vi "CumplimientoTD.vi"(8 "error in (no error)":errorcluster, 11 "Prueba21_1 in":refnum<class "Prueba21.lvclass">) -> (0 "error out":errorcluster, 3 "Prueba21_1 out":refnum<class "Prueba21.lvclass">)   [LabVIEW 2019, in "Prueba21.lvclass"]
uses:
  Prueba21.lvclass
  Prueba21.lvclass/Prueba21.ctl
panel:
  out "cumpimiento":string
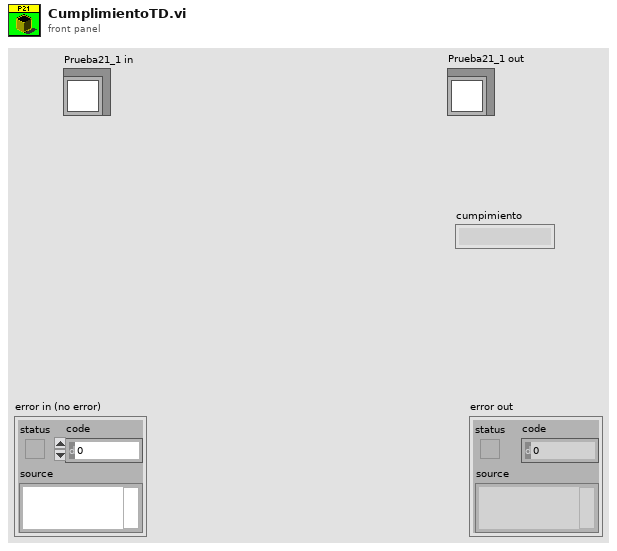
[diagram p1: front panel]
types:
  T1 = cluster{"ControlName":string, "ControlReference":refnum<vi>}[]
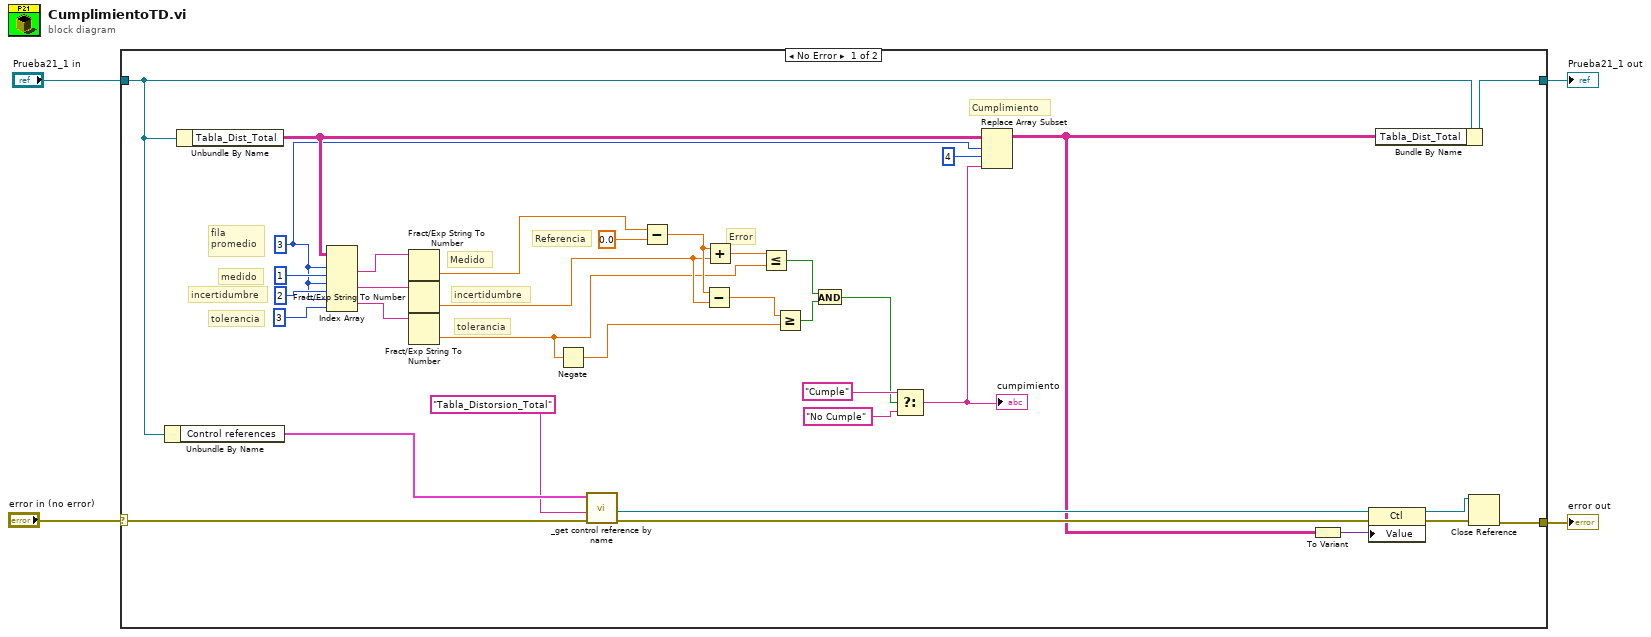
[diagram p0: block diagram]
diagram:
  n1 = case shown="No Error" "error in (no error)" {
    selector: "error in (no error)" -> [w11 w41]
    tunnel: [w13 w41] -> w3
    tunnel: [w30 w40] -> w2
    tunnel: "Prueba21_1 in" -> [w20 w40]
    frame No Error {
      w25 = 3 ("index (row)")
      # "tolerancia"
      # "incertidumbre"
      # "Medido"
      # "Referencia"
      # "tolerancia"
      # "incertidumbre"
      # "medido"
      # "fila\npromedio"
      # "Cumplimiento"
      # "Error"
      n2 = Unbundle By Name(w20) -> ("Control references"=w19:T1)
      n3 = Unbundle By Name(w20) -> ("Tabla_Dist_Total"=w28:string[][])
      n4 = Index Array(array=w28, index (row) #1=w25, index (col) #1=1 ("disabled index (col)"), index (row) #2=w25, index (col) #2=2 ("disabled index (col)"), index (row) #3=w25, index (col) #3=3 ("disabled index (col)")) -> (element #1=w9:string, element #2=w8:string, element #3=w7:string)
      n5 = Fract/Exp String To Number(string=w9) -> (number=w24:dbl)  [unwired: 3 in, 1 out]
      n6 = Fract/Exp String To Number(string=w8) -> (number=w23:dbl)  [unwired: 3 in, 1 out]
      n7 = Fract/Exp String To Number(string=w7) -> (number=w21:dbl)  [unwired: 3 in, 1 out]
      n8 = Negate(x=w21) -> (-x=w22:dbl)
      n9 = call "_get control reference by name.vi"("error in (no error)"=w11, "Control name"="Tabla_Distorsion_Total", "Control references"=w19) -> ("error out"=w12:errorcluster, "Ctl Refnum"=w17:refnum<vi>)  [unwired: 3 in]
      n10 = Subtract(x=w24, y=0.0) -> (x-y=w31:dbl)
      n11 = Subtract(x=w31, y=w23) -> (x-y=w36:dbl)
      n12 = Add(x=w31, y=w23) -> (x+y=w39:dbl)
      n13 = Less Or Equal?(x=w39, y=w21) -> (x <= y?=w38:bool)
      n14 = Greater Or Equal?(x=w36, y=w22) -> (x >= y?=w37:bool)
      n15 = And(x=w38, y=w37) -> (x .and. y?=w6:bool)
      n16 = Select(t="Cumple", s=w6, f="No Cumple") -> (s? t:f=w33:string)
      "cumpimiento" <- w33
      n17 = Replace Array Subset(array=w28, new element=w33, index (row)=w25, index (col)=4 ("index (row)")) -> (w5:string[][])
      n18 = To Variant(anything=w5) -> (Variant=w16:variant)
      n19 = property on="Property Node" class="Ctl"(reference=w17, error in=w12, "Value"=w16) -> (reference out=w15:refnum<vi>, error out=w14:errorcluster)
      n20 = Bundle By Name(cluster=w20, "Tabla_Dist_Total"=w5) -> (w30:refnum<class "Prueba21.lvclass">)
      n21 = Close Reference(reference=w15, error in (no error)=w14) -> (error out=w13:errorcluster)
    }
    frame Error {
    }
  }
  "error out" <- w3
  "Prueba21_1 out" <- w2
